vi "Clear MethodsCalled.vi"(8 "error in (no error)":errorcluster, 11 "MockListImp in":refnum<class "ListImp_RefSpy.lvclass">) -> (0 "error out":errorcluster, 3 "MockListImp out":refnum<class "ListImp_RefSpy.lvclass">)   [LabVIEW 2013, in "ListImp_RefSpy.lvclass"]
uses:
  ListImp_RefSpy.lvclass
  RefnumGlobal.vi
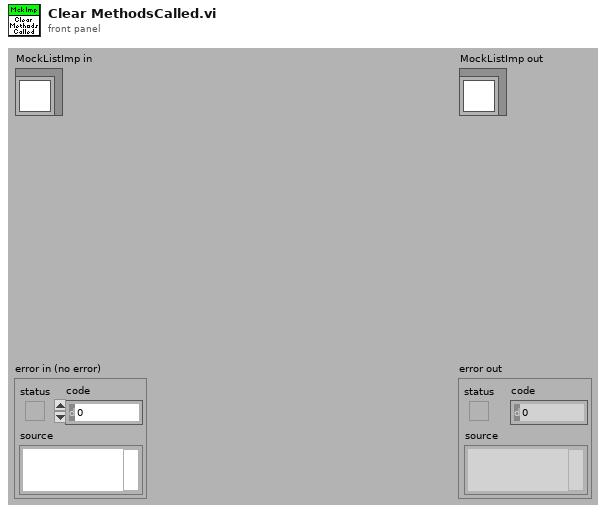
[diagram p1: front panel]
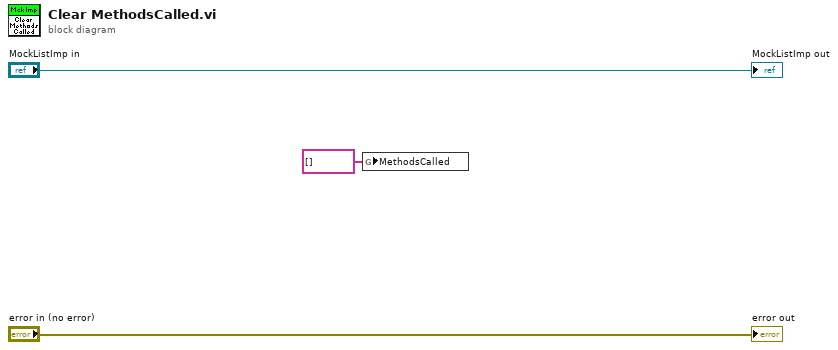
[diagram p0: block diagram]
diagram:
  n1 = global write "RefnumGlobal.vi" "MethodsCalled"(string[] [] ("MethodsCalled")) -> ()
  "error out" <- "error in (no error)"
  "MockListImp out" <- "MockListImp in"
